vi "rs3 query sensors.vi"(8 "error in (no error)":errorcluster, 11 "device in":u64) -> (0 "error out":errorcluster, 1 "error":u64, 3 "sensor_list":u64)   [LabVIEW 2017, in "libRealSense3.lvlib"]
doc: "Each DEVICE has multiple SENSORS. This call will return the handle to the array of sensors."
uses:
  <vilib>/addons/RealSense/libRealSense3.lvlib
  <vilib>/addons/RealSense/realsense-d.dll
panel:
  # "RS3 Query Sensors"
  # "(C) Intel Corp 2017.,  AGJ"
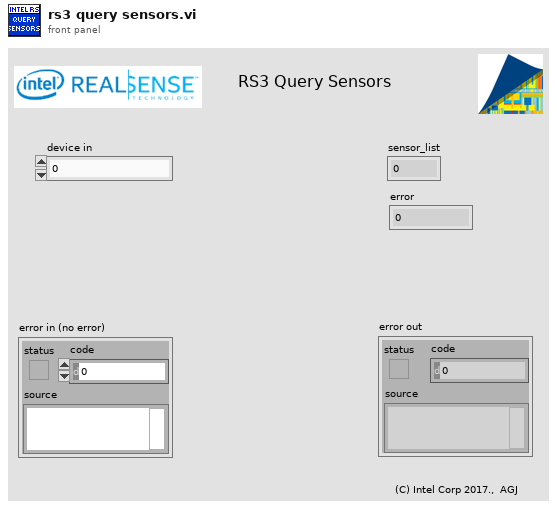
[diagram p1: front panel]
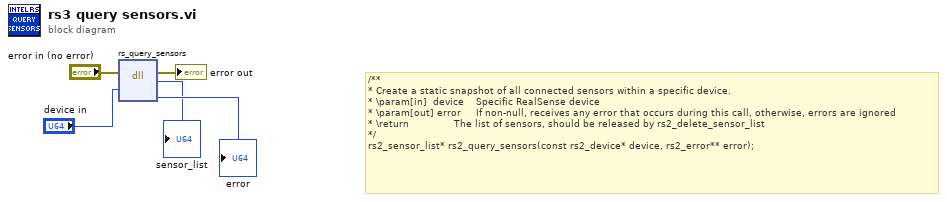
[diagram p0: block diagram]
diagram:
  # "/**\n* Create a static snapshot of all connected sensors within a specific device.\n* \\param[in]  device    Specific RealSense device\n* \\param[out] error     If non-null, receives any error that occurs during this call, otherwise, errors are ignored\n* \\return               The list of sensors, should be released by rs2_delete_sensor_list\n*/\nrs2_sensor_list* rs2_query_sensors(const rs2_device* device, rs2_error** error);"
  n1 = dll-call lib="C:/Program Files (x86)/National Instruments/LabVIEW 2017/vi.lib/addons/RealSense/realsense-d.dll" fn="rs_query_sensors"(error in="error in (no error)", "device in"="device in") -> (error out=→"error out":errorcluster, "sensor_list"=→"sensor_list":u32, "error"=→"error":u64)  [unwired: 4 in, 1 out]
